vi "Set and Save RC Config.vi"(8 "Error In":errorcluster, 10 "Aircraft RC Data":T1, 11 "Aircraft Index":u8) -> (0 "Error Out":errorcluster)   [LabVIEW 2014]
uses:
  Controls/Aircraft RC Data.ctl
  <vilib>/Utility/xml.llb/Write to XML File(string).vi
  Set Aircraft RC.vi
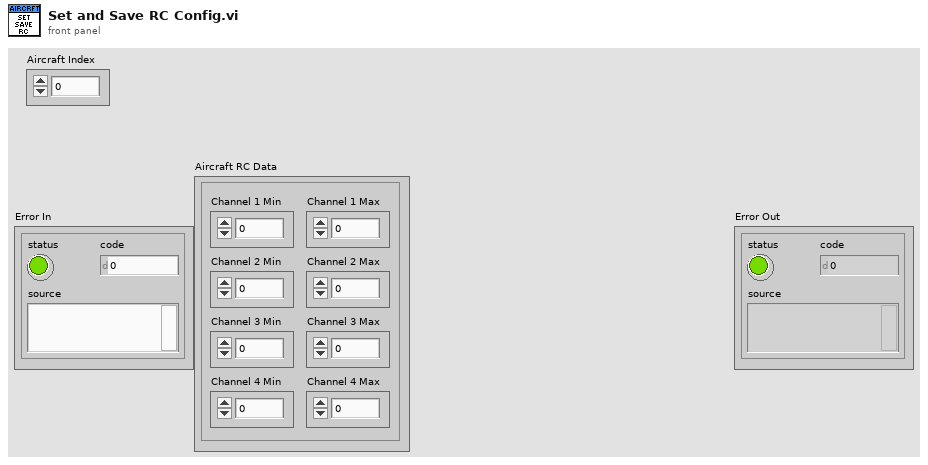
[diagram p1: front panel]
types:
  T1 = typedef "Aircraft RC Data.ctl" = cluster{"Channel 1 Min":i16, "Channel 1 Max":i16, "Channel 2 Min":i16, "Channel 2 Max":i16, "Channel 3 Min":i16, "Channel 3 Max":i16, "Channel 4 Min":i16, "Channel 4 Max":i16}
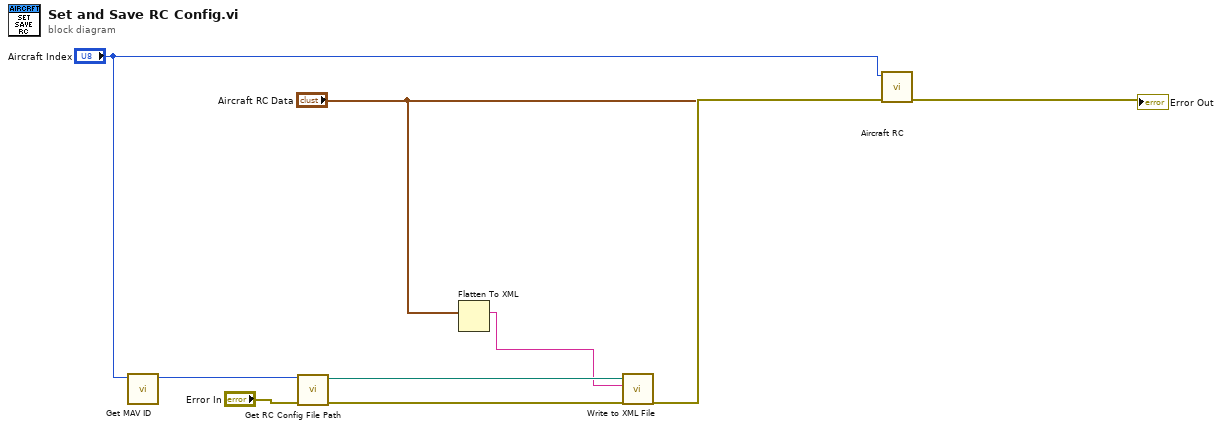
[diagram p0: block diagram]
diagram:
  n1 = call "Get MAV ID.vi"("Aircraft Index"="Aircraft Index") -> ("Aircraft ID"=w2:u8)  [unwired: 9 in, 1 out]
  n2 = call "Get RC Config File Path.vi"("Error In"="Error In", "Aircraft ID"=w2) -> ("Error Out"=w8:errorcluster, "Anchor Config File Path"=w7:path)  [unwired: 8 in]
  n3 = Flatten To XML(anything="Aircraft RC Data") -> (xml string=w3:string)
  n4 = call-poly <vilib>:"Write to XML File.vi"("error in (no error)"=w8, "XML Input"=w3, "XML File Path"=w7) -> ("error out"=w6:errorcluster)  [unwired: 6 in, 2 out]
  n5 = call-poly "Aircraft RC.vi"("Error In"=w6, "Aircraft RC Data"="Aircraft RC Data", "Aircraft ID"="Aircraft Index") -> ("Error Out"=→"Error Out":errorcluster)  [unwired: 8 in]
